vi "CSM - Read All Variable Names.vi"(5 "Permanent Variables Only? (F)":bool, 7 "error in (no error)":errorcluster) -> (1 "error out":errorcluster, 3 "All Variable Names":string[](array[string]))   [LabVIEW 2017, in "INI-Static-Variable-Support.lvlib"]
doc: "Reads all variable names currently in memory.\n\n-- <b>Controls</b> --\n- <b>Permanent Variables Only? (F)</b>: Whether to read only permanent variables.\n\n-- <b>Indicators</b> --\n- <b>All Variable Names</b>: Array of variable names."
uses:
  INI-Static-Variable-Support.lvlib
  _fgv-oper.ctl
  <userlib>/_NEVSTOP/Communicable State Machine(CSM)/_Support/ChangeFlag/ChangeFlag-Read.vi
  <userlib>/_NEVSTOP/Communicable State Machine(CSM)/_Support/ChangeFlag/ChangeFlagDB.vi
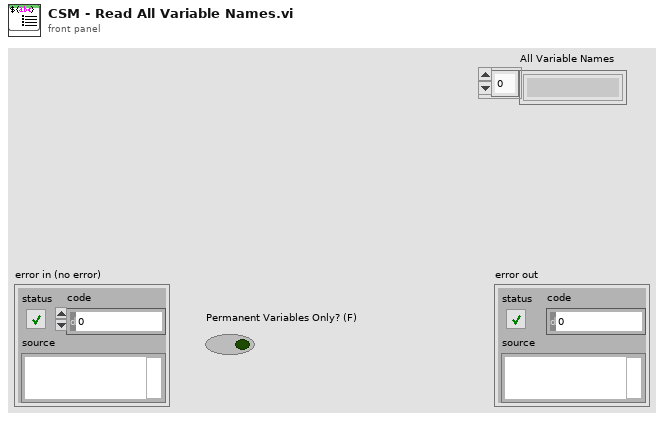
[diagram p1: front panel]
types:
  T1 = typedef "INI-Static-Variable-Support.lvlib/_fgv-oper.ctl" = enum16{"Read", "Write", "Sync", "Sessions", "List Keys", "Load", "List Files", "List Variables", "List Permanent Variables", "Mark Temp Variable as Permenent", "unload", "INIConfig(Memory)", "Reset", "Restore Variable Value"}
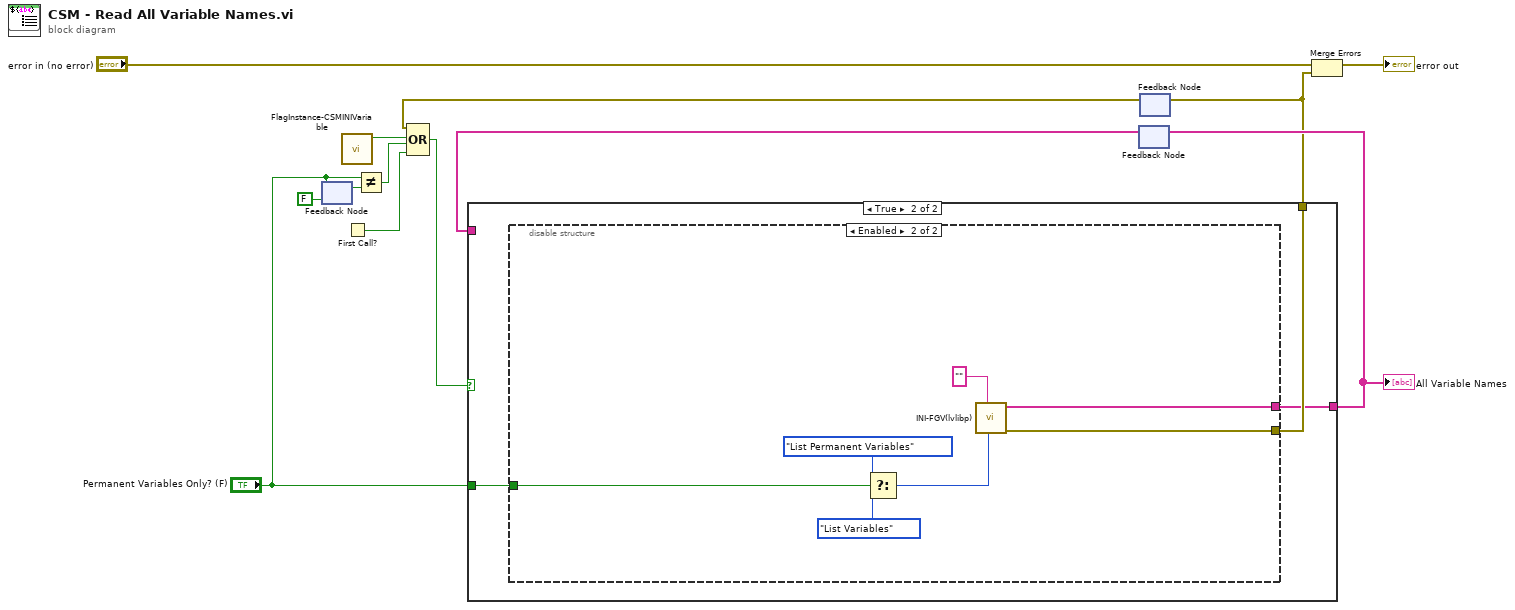
[diagram p0: block diagram]
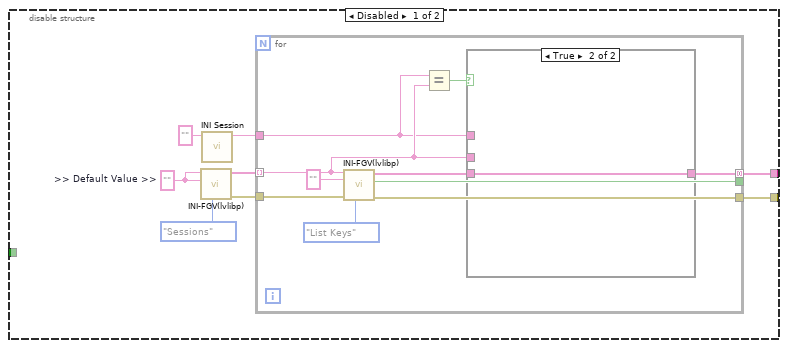
[diagram p3: hidden frame]
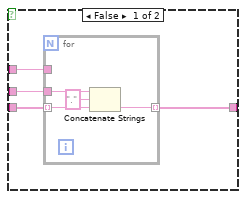
[diagram p4: hidden frame]
diagram:
  n1 = feedback #1(FALSE ("Permanent Variables Only?")) -> (w6:bool)
  n2 = feedback-in #1("Permanent Variables Only? (F)") -> ()
  n3 = call "FlagInstance-CSMINIVariable.vi"() -> ("Changed"=w1:bool)  [unwired: 10 in, 1 out]
  n4 = First Call?() -> (First Call?: T/F=w2:bool)
  n5 = Not Equal?(x="Permanent Variables Only? (F)", y=w6) -> (x != y?=w4:bool)
  n6 = feedback #2() -> (w10:string[])  [unwired: 1 in]
  n7 = feedback #3() -> (w8:errorcluster)  [unwired: 1 in]
  n8 = Compound Arithmetic op=OR(w8, w1, w4, w2) -> (w7:bool)
  n9 = case shown="True" w7 {
    tunnel: [_ w17] -> w9
    tunnel: [w14 w16] -> w11
    tunnel: w10 -> [w14 _]
    tunnel: "Permanent Variables Only? (F)" -> [_ w15]
    frame False {
    }
    frame True {
      n10 = disable-structure shown="Enabled" {
        disable-tunnel: [w25 w50] -> w17
        disable-tunnel: [w24 w51] -> w16
        disable-tunnel: w15 -> [_ w46]
        frame Disabled {
          w22 = ""  # >> Default Value >>
          n11 = call "INI-FGV(lvlibp).vi"("Enum"=_fgv-oper."Sessions", ">> Default Value >>"=w22, ">> Variable Name >>"=w22) -> ("error out"=w20:errorcluster, "Array"=w21:string[])  [unwired: 5 in, 2 out]
          n12 = call "INI Session.vi"("Section Name(\"\" as Default)"="" ("Section Name(\"\" as Default)")) -> ("App.Name"=w18:string)  [unwired: 10 in]
          n13 = for {
            tunnel: [w34] -> w25
            tunnel: [w29] -> w24 mode=concatenating
            tunnel: [w33] -> _
            tunnel: w21 -> [w28] mode=indexing
            tunnel: w20 -> [w31]
            tunnel: w18 -> [w27]
            n14 = call "INI-FGV(lvlibp).vi"("Enum"=_fgv-oper."List Keys", "error IN"=w31, ">> Default Value >>"="", ">> Variable Name >>"=w28) -> ("error out"=w34:errorcluster, "Key?"=w33:bool, "Array"=w30:string[])  [unwired: 4 in, 1 out]
            n15 = Equal?(x=w27, y=w28) -> (x = y?=w26:bool)
            n16 = case shown="True" w26 {
              tunnel: w30 -> [w39 w44]
              tunnel: [w38 w44] -> w29
              tunnel: w28 -> [w37 _]
              tunnel: w27 -> [w36 _]
              frame False {
                n17 = for {
                  tunnel: w39 -> [w43] mode=indexing
                  tunnel: w37 -> [w42]
                  tunnel: [w40] -> w38 mode=indexing
                  tunnel: w36 -> [_]
                  n18 = Concatenate Strings(w42, "." ("string"), w43) -> (w40:string)
                }
              }
              frame True {
              }
            }
          }
        }
        frame Enabled {
          n19 = Select(t=_fgv-oper."List Permanent Variables" ("Enum"), s=w46, f=_fgv-oper."List Variables" ("Enum")) -> (s? t:f=w47:T1)
          n20 = call "INI-FGV(lvlibp).vi"("Enum"=w47, "Prefered Section"="") -> ("error out"=w50:errorcluster, "Array"=w51:string[])  [unwired: 6 in, 2 out]
        }
      }
    }
  }
  "All Variable Names" <- w11
  n21 = feedback-in #2(w11) -> ()
  n22 = feedback-in #3(w9) -> ()
  n23 = Merge Errors("error in (no error)", w9) -> (→"error out":errorcluster)
